vi "drop-test.vi"() -> ()   [LabVIEW 2010]
uses:
  <vilib>/Utility/miscctls.llb/LVPoint32TypeDef.ctl
  <vilib>/Utility/inputDevices.llb/mouseAcquire.vi
  shell32.dll
  user32.dll
panel:
  out "file count":u32
  out "Array":string[](array[string])
  out "Innerhalb der Grenzen?":bool
  in  "Boolesch":bool
  out "Zeile":i32
  in  "Listenfeld":i32(listbox)
  in  "Numerisch":dbl
  out "win msg queue":T1
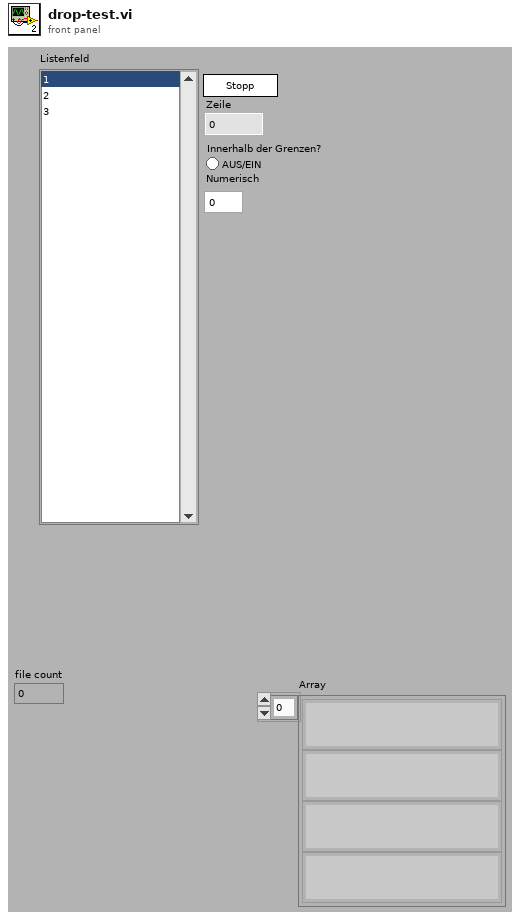
[diagram p1: front panel]
types:
  T1 = typedef "Win Msg Queue RefNum" = refnum<k1>
  T2 = typedef "LVPoint32TypeDef.ctl" = cluster{"Horizontal":i32, "Vertical":i32}
  T3 = cluster{"Horizontal":i32, "Vertical":i32, "Scrolling":i32}
  T4 = cluster{"hWnd":u32, "Msg":u32, "wParam":u32, "lParam":i32, "time":u32, "point":cluster{"X":i32, "Y":i32}}
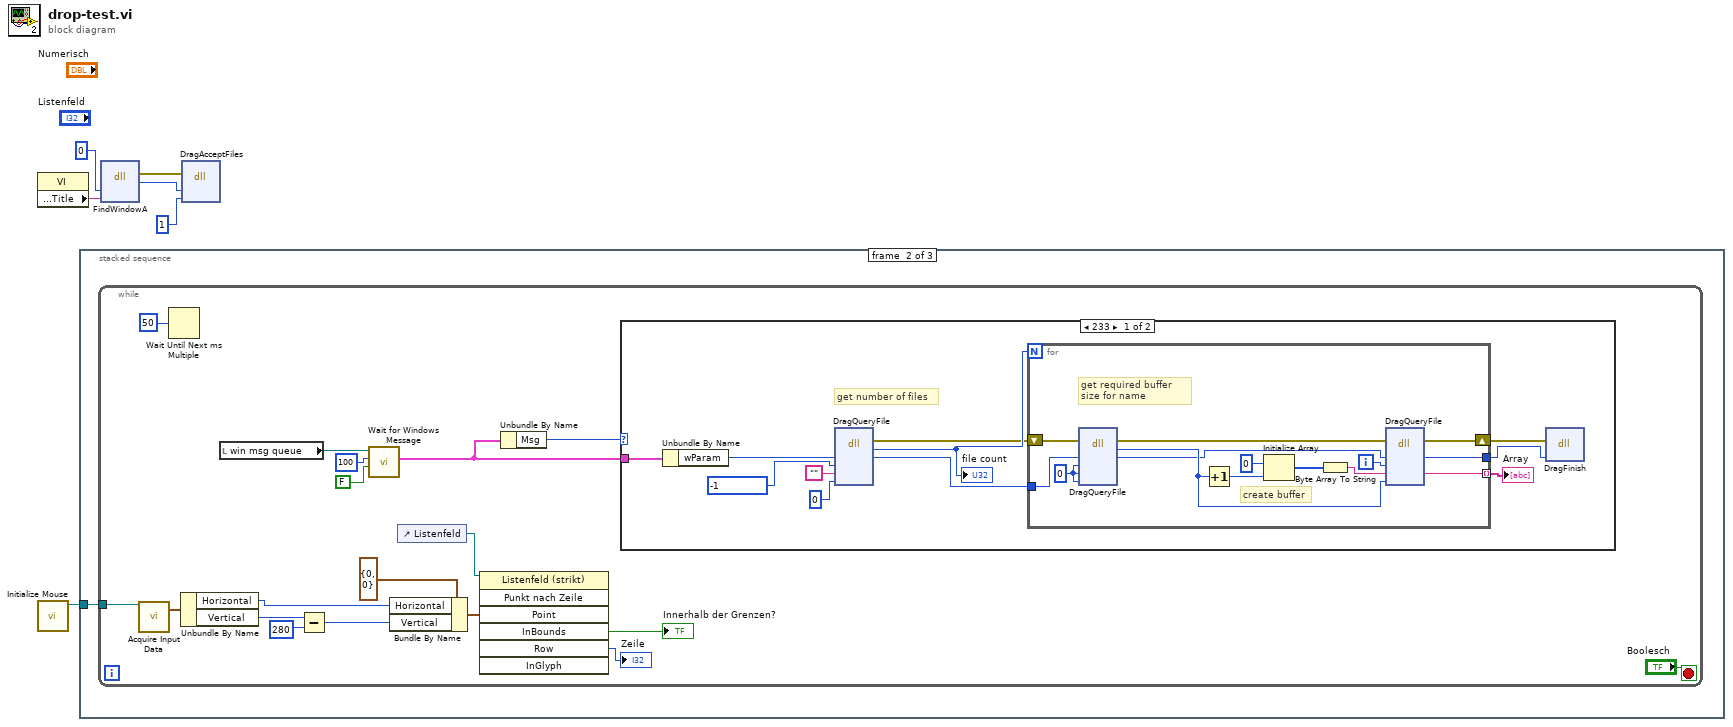
[diagram p0: block diagram]
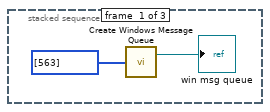
[diagram p2: hidden frame]
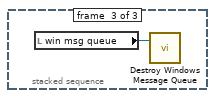
[diagram p4: hidden frame]
diagram:
  n1 = property class="VI"() -> ("Front Panel Window:Title"=w5:string)  [unwired: 2 in, 2 out]
  n2 = call <vilib>:"Initialize Mouse.vi"() -> ("device ID"=w1:refnum<k1>)  [unwired: 10 in, 1 out]
  n3 = stacked-sequence {
    tunnel: w1 -> [_ w9 _]
    frame #0 {
      n4 = call <userlib>:"Create Windows Message Queue.vi"("Messeges (none)"=u32[] [563]) -> ("win msg queue"=→"win msg queue":T1)  [unwired: 2 in, 1 out]
    }
    frame #1 {
      n5 = while {
        tunnel: w9 -> [w25]
        stop <- "Boolesch" stop-if-true
        n6 = call-poly <vilib>:"Acquire Input Data.vi"("device ID"=w25) -> ("axis info"=w24:T3)  [unwired: 15 in, 3 out]
        n7 = Wait Until Next ms Multiple(millisecond multiple=u32 50 ("Vielfache von ms")) -> ()  [unwired: 1 out]
        n8 = Unbundle By Name(w24) -> ("Horizontal"=w19:i32, "Vertical"=w13:i32)
        n9 = local read "win msg queue"() -> (w23:T1)
        n10 = Subtract(x=w13, y=280) -> (x-y=w14:i32)
        n11 = call <userlib>:"Wait for Windows Message.vi"("win msg queue"=w23, "ms timeout (-1)"=100, "ignore previous (F)"=FALSE ("ignore previous (T)")) -> ("Message"=w10:T4)  [unwired: 1 in, 5 out]
        n12 = Bundle By Name(cluster=T2 {"Horizontal"=0, "Vertical"=0} ("Koordinaten"), "Horizontal"=w19, "Vertical"=w14) -> (w17:T2)
        n13 = control-ref of="Listenfeld"() -> (w18:refnum<vi>)
        n14 = invoke class="Listenfeld (strikt)" method="Punkt nach Zeile"(reference=w18, "Point"=w17) -> ("InBounds"=→"Innerhalb der Grenzen?":bool, "Row"=→"Zeile":i32)  [unwired: 5 in, 5 out]
        n15 = Unbundle By Name(w10) -> ("Msg"=w11:u32)
        n16 = case shown="233" w11 {
          tunnel: w10 -> [w38 _]
          frame 563 {
            # "get number of files"
            n17 = Unbundle By Name(w38) -> ("wParam"=w37:u32)
            n18 = dll-call lib="shell32.dll" fn="DragQueryFile"("hDrop"=w37, "iFile"=-1, "lpszFile"="", "cch"=0) -> (error out=w34:errorcluster, "return type"=w35:u32, "hDrop"=w33:i32)  [unwired: 6 in, 1 out]
            "file count" <- w35
            n19 = for {
              N: w35 -> [_]
              shift-right: [w41] -> w32
              shift-left: w34 -> [w52]
              tunnel: w33 -> [w51]
              tunnel: [w42] -> w31
              tunnel: [w39] -> w28 mode=indexing
              i -> [w44]
              w48 = 0
              # "create buffer"
              # "get required buffer size for name"
              n20 = dll-call lib="shell32.dll" fn="DragQueryFile"(error in=w52, "hDrop"=w51, "iFile"=w48, "lpszFile"=w48, "cch"=w48) -> (error out=w40:errorcluster, "return type"=w45:u32, "hDrop"=w43:i32)  [unwired: 5 in, 1 out]
              n21 = Increment(x=w45) -> (x+1=w47:u32)
              n22 = Initialize Array(u8 0, w47) -> (w50:u8[])
              n23 = Byte Array To String(unsigned byte array=w50) -> (string=w46:string)
              n24 = dll-call lib="shell32.dll" fn="DragQueryFile"(error in=w40, "hDrop"=w43, "iFile"=w44, "lpszFile"=w46, "cch"=w45) -> (error out=w41:errorcluster, "hDrop"=w42:i32, "lpszFile"=w39:string)  [unwired: 5 in, 1 out]
            }
            "Array" <- w28
            n25 = dll-call lib="shell32.dll" fn="DragFinish"(error in=w32, "hDrop"=w31) -> ()  [unwired: 4 in, 2 out]
          }
          frame 0, Default {
            # "Do nothing\nThis case is executed if the wait times out\n(It returns Msg 0)."
          }
        }
      }
    }
    frame #2 {
      n26 = local read "win msg queue"() -> (w53:T1)
      n27 = call <userlib>:"Destroy Windows Message Queue.vi"("win msg queue"=w53) -> ()  [unwired: 1 in, 1 out]
    }
  }
  n28 = dll-call lib="user32.dll" fn="FindWindowA" label="FindWindow"("lpszClassName"=0, "lpszWindowName"=w5) -> (error out=w6:errorcluster, "hWnd"=w2:u32)  [unwired: 5 in, 1 out]
  n29 = dll-call lib="shell32.dll" fn="DragAcceptFiles"(error in=w6, "hWnd"=w2, "fAccept"=1) -> ()  [unwired: 5 in, 2 out]
